vi "User_Defined_Test_Test_XML_012.vi"() -> (3 "Unit Test Framework Results":T1)   [LabVIEW 2014, in "XML_Deserializer.lvlib"]
doc: "Use this template to create a user-defined test VI. Define your test requirements and wire the results to the <b>Result (Test)</b> control. Do not modify the <b>Unit Test Framework Results</b> indicator."
uses:
  XML VIs/API/XML_Deserializer.lvlib
  <vilib>/utf/common/utf_test_result_troll.ctl
  <vilib>/utf/common/utf_test_result.ctl
  <vilib>/utf/common/utf_test_result_failure.ctl
  <vilib>/utf/common/utf_test_comparison_operators.ctl
  <vilib>/utf/common/utf_vi_tag.ctl
  XML VIs/API/Controls/Modbus_Items.ctl
  XML VIs/API/Controls/Modbus_Item_Type.ctl
  <vilib>/utf/NI_UnitTestFramework.lvlib
  Shared/Modbus Shared.lvlib
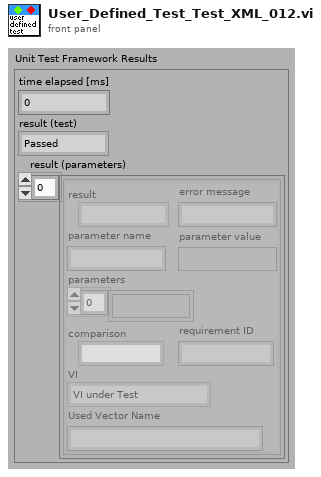
[diagram p1: front panel]
types:
  T1 = typedef "NI_UnitTestFramework.lvlib/utf_test_result_troll.ctl" = cluster{"time elapsed [ms]":u32, "result (test)":T2, "result (parameters)":T3[]}
  T2 = typedef "NI_UnitTestFramework.lvlib/utf_test_result.ctl" = enum16{"Passed", "Failed", "Error", "Skipped", "Not Processed"}
  T3 = typedef "NI_UnitTestFramework.lvlib/utf_test_result_failure.ctl" = cluster{"result":T2, "error message":string, "parameter name":string, "parameter value":variant, "parameters":variant[], "comparison":T4, "requirement ID":string, "VI":T5, "Used Vector Name":string}
  T4 = typedef "NI_UnitTestFramework.lvlib/utf_test_comparison_operators.ctl" = enum16{"=", "!=", ">", ">=", "<", "<=", "range", "symmetric tolerance", "asymmetric tolerance", "string contains", "string not contain", "array size", "string length", "array range", "by element", "array range (limit array)", "user-defined", "array contains", "array not contain", "vector length", "= (elm)", "!= (elm)", "= (case insensitive)", "!= (case insensitive)"}
  T5 = typedef "NI_UnitTestFramework.lvlib/utf_vi_tag.ctl" = enum16{"Setup VI", "VI under Test", "Teardown VI"}
  T6 = typedef "Modbus Shared.lvlib/Modbus_Items.ctl" = cluster{"Modbus Type":T7, "Base Name":string, "Starting Address":u16, "Quantity":u16}
  T7 = typedef "Modbus Shared.lvlib/Modbus_Item_Type.ctl" = enum16{"Read Coils", "Read Discrete Inputs", "Read Holding Registers", "Read Input Registers", "Write Multiple Coils", "Write Multiple Holding Registers", "Write Single Coil", "Write Single Holding Register", "Write Multiple Discrete Inputs", "Write Multiple Input Registers"}
  T8 = cluster{"Communication_Type":i32, "Modbus_Type":i32, "Read_Write_Loop_Period":i64, "TCP Settings":cluster{"TCP_Settings_Port":u16, "TCP_Settings_IP_Timeout":u32, "TCP_Settings_IP_Slave_Address":string}, "Serial Settings":cluster{"Serial_Settings_Flow_Control":i32, "Serial_Settings_Baud_Rate":u32, "Serial_Settings_Parity":i32, "Serial_Settings_Resource_Name":string, "Serial_Settings_Serial_Type":i32, "Serial_Settings_Unit_ID":i8}}
  T9 = cluster{"status":bool, "code":bool, "source":bool}
  T10 = cluster{"Communication_Type":bool, "Modbus_Type":bool, "Read_Write_Loop_Period":bool, "TCP Settings":cluster{"TCP_Settings_Port":bool, "TCP_Settings_IP_Timeout":bool, "TCP_Settings_IP_Slave_Address":bool}, "Serial Settings":cluster{"Serial_Settings_Flow_Control":bool, "Serial_Settings_Baud_Rate":bool, "Serial_Settings_Parity":bool, "Serial_Settings_Resource_Name":bool, "Serial_Settings_Serial_Type":bool, "Serial_Settings_Unit_ID":bool}}
  T11 = cluster{"Modbus Type":bool, "Base Name":bool, "Starting Address":bool, "Quantity":bool}[]
  T12 = cluster{"TCP_Settings_Port":bool, "TCP_Settings_IP_Timeout":bool, "TCP_Settings_IP_Slave_Address":bool}
  T13 = cluster{"Serial_Settings_Flow_Control":bool, "Serial_Settings_Baud_Rate":bool, "Serial_Settings_Parity":bool, "Serial_Settings_Resource_Name":bool, "Serial_Settings_Serial_Type":bool, "Serial_Settings_Unit_ID":bool}
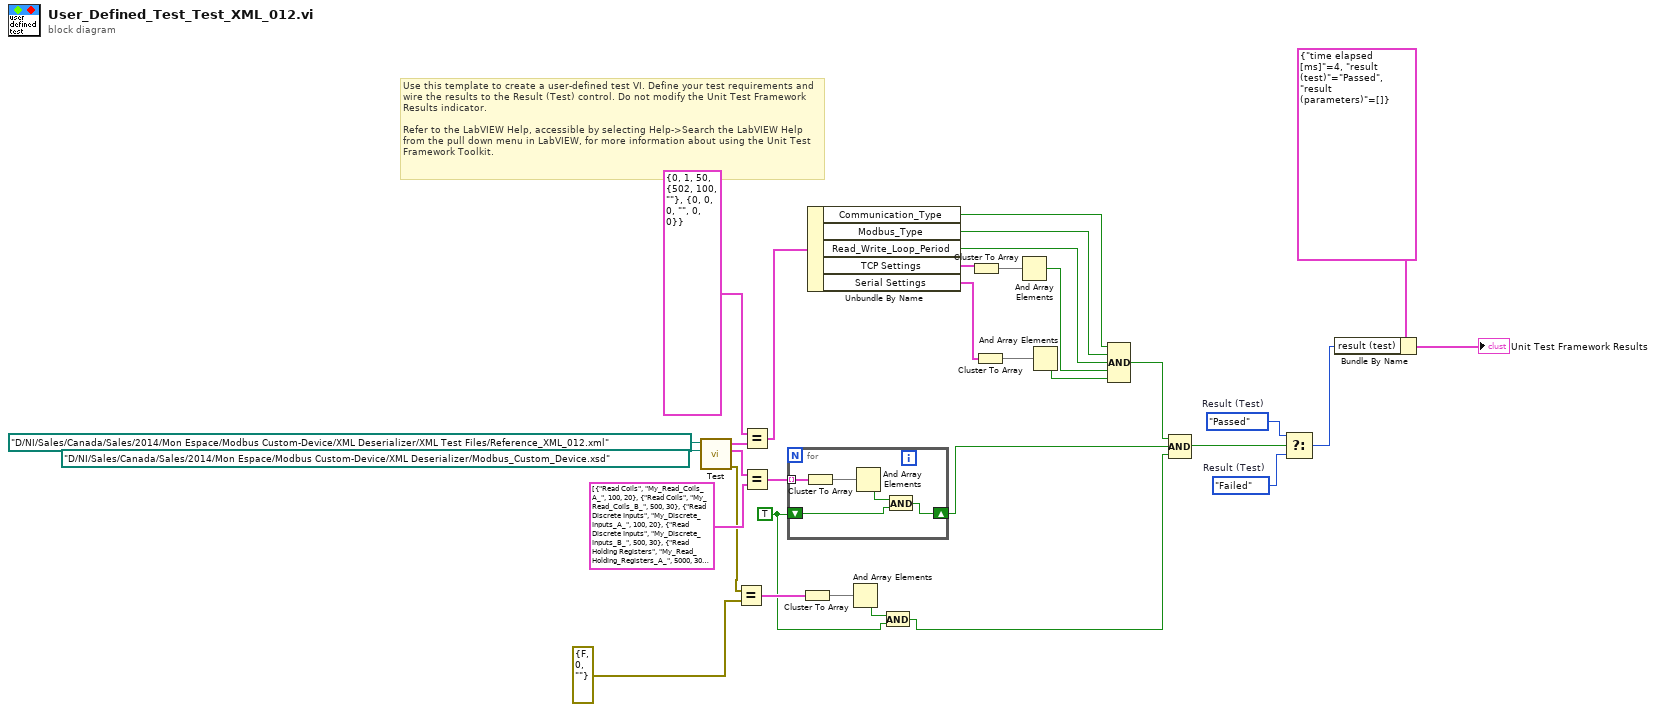
[diagram p0: block diagram]
diagram:
  w15 = utf_test_result."Failed"  # Result (Test)
  w12 = TRUE
  w16 = utf_test_result."Passed"  # Result (Test)
  # "Use this template to create a user-defined test VI. Define your test requirements and wire the results to the Result (Test) control. Do not modify the Unit Test Framework Results indicator. \n\nRefer to the LabVIEW Help, accessible by selecting Help->Search the LabVIEW Help from the pull down menu in LabVIEW, for more information about using the Unit Test Framework Toolkit."
  n1 = call "Test.vi"("XSD File Path"=path "D:/NI/Sales/Canada/Sales/2014/Mon Espace/Modbus Custom-Device/XML Deserializer/Modbus_Custom_Device.xsd", "XML File Path"=path "D:/NI/Sales/Canada/Sales/2014/Mon Espace/Modbus Custom-Device/XML Deserializer/XML Test Files/Reference_XML_012.xml") -> ("error out"=w21:errorcluster, "List of Modbus Items"=w26:T6[], "General Settings"=w28:T8)  [unwired: 7 in]
  n2 = Equal?(x=w21, y=errorcluster {"status"=FALSE, "code"=0, "source"=""} ("error out")) -> (x = y?=w20:T9)
  n3 = Equal?(x=T8 {"Communication_Type"=0, "Modbus_Type"=1, "Read_Write_Loop_Period"=50, "TCP Settings"={"TCP_Settings_Port"=502, "TCP_Settings_IP_Timeout"=100, "TCP_Settings_IP_Slave_Address"=""}, "Serial Settings"={"Serial_Settings_Flow_Control"=0, "Serial_Settings_Baud_Rate"=0, "Serial_Settings_Parity"=0, "Serial_Settings_Resource_Name"="", "Serial_Settings_Serial_Type"=0, "Serial_Settings_Unit_ID"=0}} ("General Settings"), y=w28) -> (x = y?=w18:T10)
  n4 = Equal?(x=w26, y=T6[] [{"Modbus Type"=enum."Read Coils", "Base Name"="My_Read_Coils_A_", "Starting Address"=100, "Quantity"=20}, {"Modbus Type"=enum."Read Coils", "Base Name"="My_Read_Coils_B_", "Starting Address"=500, "Quantity"=30}, {"Modbus Type"=enum."Read Discrete Inputs", "Base Name"="My_Discrete_Inputs_A_", "Starting Address"=100, "Quantity"=20}, {"Modbus Type"=enum."Read Discrete Inputs", "Base Name"="My_Discrete_Inputs_B_", "Starting Address"=500, "Quantity"=30}, {"Modbus Type"=enum."Read Holding Registers", "Base Name"="My_Read_Holding_Registers_A_", "Starting Address"=5000, "Quantity"=30}, {"Modbus Type"=enum."Read Holding Registers", "Base Name"="My_Read_Holding_Registers_B_", "Starting Address"=1500, "Quantity"=30}, {"Modbus Type"=enum."Read Holding Registers", "Base Name"="My_Read_Holding_Registers_C_", "Starting Address"=5000, "Quantity"=30}, {"Modbus Type"=enum."Read Input Registers", "Base Name"="My_Read_Input_Registers_A_", "Starting Address"=5000, "Quantity"=30}, {"Modbus Type"=enum."Read Input Registers", "Base Name"="My_Read_Input_Registers_B_", "Starting Address"=1500, "Quantity"=30}, {"Modbus Type"=enum."Read Input Registers", "Base Name"="My_Read_Input_Registers_C_", "Starting Address"=5000, "Quantity"=30}, {"Modbus Type"=enum."Write Multiple Coils", "Base Name"="My_Write_Multiple_Coils_A", "Starting Address"=0, "Quantity"=6000}, {"Modbus Type"=enum."Write Multiple Holding Registers", "Base Name"="My_Write_Multiple_Holding_Registers_A", "Starting Address"=7000, "Quantity"=30}, {"Modbus Type"=enum."Write Multiple Input Registers", "Base Name"="My_Write_Multiple_Input_Registers_A", "Starting Address"=8000, "Quantity"=30}, {"Modbus Type"=enum."Write Single Coil", "Base Name"="My_Write_Single_Coil_A", "Starting Address"=9000, "Quantity"=1}, {"Modbus Type"=enum."Write Single Holding Register", "Base Name"="My_Write_Single_Holding_Register_A", "Starting Address"=10000, "Quantity"=1}, {"Modbus Type"=enum."Write Multiple Discrete Inputs", "Base Name"="My_Write_Multiple_Discrete_Input_A", "Starting Address"=11000, "Quantity"=30}] ("List of Modbus Items")) -> (x = y?=w24:T11)
  n5 = for {
    tunnel: w24 -> [w37] mode=indexing
    shift-right: [w33] -> w23
    shift-left: w12 -> [w34]
    n6 = Cluster To Array(cluster=w37) -> (array=w36:bool[])
    n7 = And Array Elements(Boolean array=w36) -> (logical AND=w35:bool)
    n8 = And(x=w35, y=w34) -> (x .and. y?=w33:bool)
  }
  n9 = Cluster To Array(cluster=w20) -> (array=w2:bool[])
  n10 = Unbundle By Name(w18) -> ("Communication_Type"=w3:bool, "Modbus_Type"=w4:bool, "Read_Write_Loop_Period"=w5:bool, "TCP Settings"=w7:T12, "Serial Settings"=w8:T13)
  n11 = And Array Elements(Boolean array=w2) -> (logical AND=w1:bool)
  n12 = And(x=w1, y=w12) -> (x .and. y?=w19:bool)
  n13 = Cluster To Array(cluster=w7) -> (array=w9:bool[])
  n14 = Cluster To Array(cluster=w8) -> (array=w11:bool[])
  n15 = And Array Elements(Boolean array=w9) -> (logical AND=w6:bool)
  n16 = And Array Elements(Boolean array=w11) -> (logical AND=w10:bool)
  n17 = Compound Arithmetic op=AND(w3, w4, w5, w6, w10) -> (w13:bool)
  n18 = Compound Arithmetic op=AND(w13, w23, w19) -> (w17:bool)
  n19 = Select(t=w16, s=w17, f=w15) -> (s? t:f=w14:T2)
  n20 = Bundle By Name(cluster=T1 {"time elapsed [ms]"=4, "result (test)"=enum."Passed", "result (parameters)"=[]} ("Unit Test Framework - Result"), "result (test)"=w14) -> (→"Unit Test Framework Results":T1)
